vi "DoCollision.vi"(8 "error in (no error)":errorcluster, 10 "GameObject in":refnum<class "GameObject.lvclass">, 11 "Object in":refnum<class "GameObject.lvclass">) -> (0 "error out":errorcluster, 1 "Collided?":bool, 2 "GameObject out":refnum<class "GameObject.lvclass">, 3 "Object out":refnum<class "GameObject.lvclass">)   [LabVIEW 2019, in "RT_Game.lvlib" / "GameObject.lvclass"]
uses:
  GameObject.lvclass
  GameObject.lvclass/GameObject.ctl
  Globals.vi
  RT_Game.lvlib
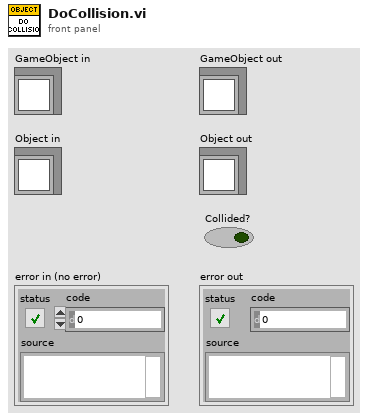
[diagram p1: front panel]
types:
  T1 = typedef "RT_Game.lvlib/Velocity.ctl" = cluster{"x":dbl, "y":dbl}
  T2 = typedef "RT_Game.lvlib/Game.lvclass/Coordinate.ctl" = cluster{"x":dbl, "y":dbl}
  T3 = typedef "RT_Game.lvlib/Direction.ctl" = enum16{"none", "Both", "left", "right", "up", "down"}
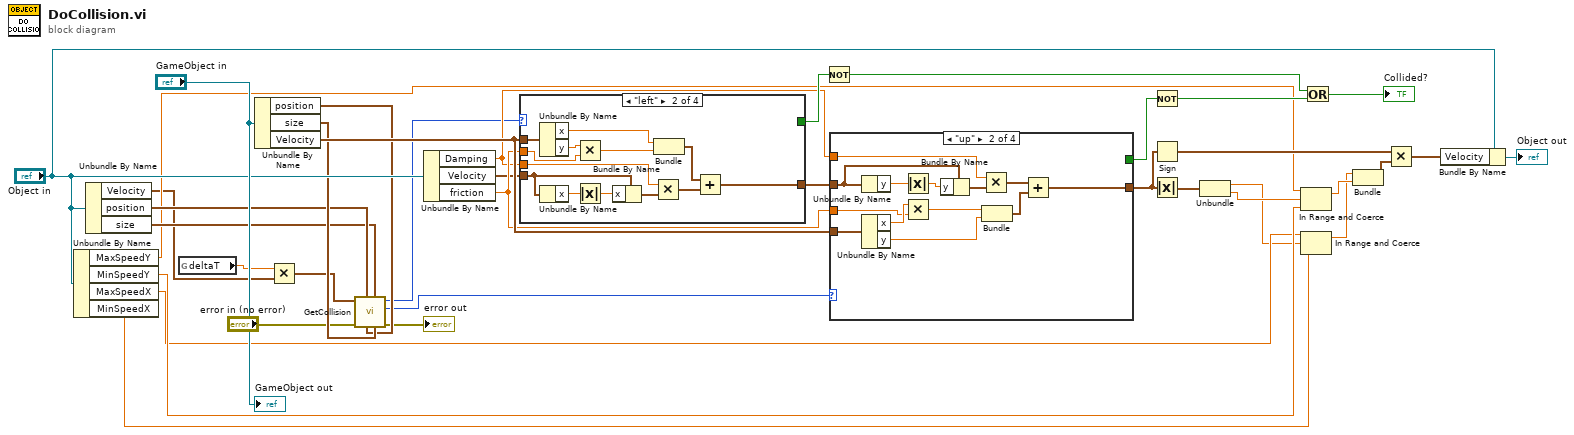
[diagram p0: block diagram]
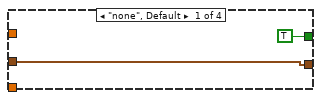
[diagram p2: hidden frame]
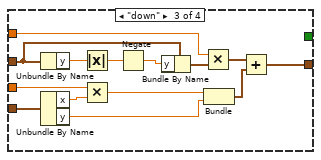
[diagram p3: hidden frame]
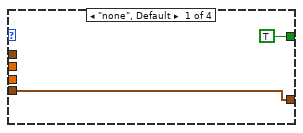
[diagram p5: hidden frame]
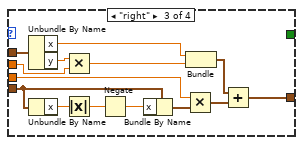
[diagram p6: hidden frame]
diagram:
  n1 = Unbundle By Name("Object in") -> ("MaxSpeedY"=w18:dbl, "MinSpeedY"=w17:dbl, "MaxSpeedX"=w6:dbl, "MinSpeedX"=w5:dbl)
  n2 = Unbundle By Name("Object in") -> ("Velocity"=w10:T1, "position"=w26:T2, "size"=w25:T2)
  n3 = global read "Globals.vi" "deltaT"() -> (w11:dbl)
  n4 = Unbundle By Name("GameObject in") -> ("position"=w27:T2, "size"=w28:T2, "Velocity"=w29:T1)
  n5 = Multiply(x=w11, y=w10) -> (x*y=w16:T1)
  n6 = call "GetCollision.vi"("TheirSize"=w28, "MySize"=w25, "TheirPosition"=w27, "MyPosition"=w26, "error in (no error)"="error in (no error)", "Velocity"=w16) -> ("error out"=→"error out":errorcluster, "direction_y"=w14:T3, "direction_x"=w13:T3)  [unwired: 3 in]
  n7 = Unbundle By Name("Object in") -> ("Damping"=w21:dbl, "Velocity"=w15:T1, "friction"=w22:dbl)
  n8 = case shown="\"left\"" w13 {
    tunnel: w15 -> [w39 w48 w62 w67]
    tunnel: [w39 w50 w64 w67] -> w23
    tunnel: w29 -> [_ w52 w66 _]
    tunnel: w21 -> [_ w44 w58 _]
    tunnel: w22 -> [_ w40 w53 _]
    tunnel: [TRUE _ _ _] -> w30
    frame "none", Default {
    }
    frame "left" {
      n9 = Unbundle By Name(w52) -> ("x"=w46:dbl, "y"=w42:dbl)
      n10 = Unbundle By Name(w48) -> ("x"=w47:dbl)
      n11 = Multiply(x=w42, y=w40) -> (x*y=w41:dbl)
      n12 = Absolute Value(x=w47) -> (abs(x)=w43:dbl)
      n13 = Bundle By Name(cluster=w48, "x"=w43) -> (w49:T1)
      n14 = Multiply(x=w44, y=w49) -> (x*y=w45:T1)
      n15 = Bundle("x"=w46, w41) -> (w51:cluster{"x":dbl, dbl})  [unwired: 1 in]
      n16 = Add(x=w51, y=w45) -> (x+y=w50:T1)
    }
    frame "right" {
      n17 = Unbundle By Name(w66) -> ("x"=w60:dbl, "y"=w55:dbl)
      n18 = Unbundle By Name(w62) -> ("x"=w61:dbl)
      n19 = Multiply(x=w55, y=w53) -> (x*y=w54:dbl)
      n20 = Absolute Value(x=w61) -> (abs(x)=w57:dbl)
      n21 = Negate(x=w57) -> (-x=w56:dbl)
      n22 = Bundle By Name(cluster=w62, "x"=w56) -> (w63:T1)
      n23 = Multiply(x=w58, y=w63) -> (x*y=w59:T1)
      n24 = Bundle("x"=w60, w54) -> (w65:cluster{"x":dbl, dbl})  [unwired: 1 in]
      n25 = Add(x=w65, y=w59) -> (x+y=w64:T1)
    }
    frame "Both" {
    }
  }
  n26 = Not(x=w30) -> (.not. x?=w34:bool)
  n27 = case shown="\"up\"" w14 {
    tunnel: w23 -> [w69 w77 w91 w97]
    tunnel: [w69 w79 w93 w97] -> w19
    tunnel: w29 -> [_ w81 w95 _]
    tunnel: w21 -> [_ w73 w86 _]
    tunnel: w22 -> [_ w71 w83 _]
    tunnel: [TRUE _ _ _] -> w31
    frame "none", Default {
    }
    frame "up" {
      n28 = Unbundle By Name(w77) -> ("y"=w78:dbl)
      n29 = Unbundle By Name(w81) -> ("x"=w72:dbl, "y"=w80:dbl)
      n30 = Absolute Value(x=w78) -> (abs(x)=w74:dbl)
      n31 = Multiply(x=w72, y=w71) -> (x*y=w70:dbl)
      n32 = Bundle By Name(cluster=w77, "y"=w74) -> (w75:T1)
      n33 = Multiply(x=w73, y=w75) -> (x*y=w76:T1)
      n34 = Bundle(w70, "y"=w80) -> (w82:cluster{dbl, "y":dbl})  [unwired: 1 in]
      n35 = Add(x=w76, y=w82) -> (x+y=w79:T1)
    }
    frame "down" {
      n36 = Unbundle By Name(w91) -> ("y"=w92:dbl)
      n37 = Unbundle By Name(w95) -> ("x"=w85:dbl, "y"=w94:dbl)
      n38 = Absolute Value(x=w92) -> (abs(x)=w88:dbl)
      n39 = Multiply(x=w83, y=w85) -> (x*y=w84:dbl)
      n40 = Negate(x=w88) -> (-x=w87:dbl)
      n41 = Bundle By Name(cluster=w91, "y"=w87) -> (w89:T1)
      n42 = Multiply(x=w86, y=w89) -> (x*y=w90:T1)
      n43 = Bundle(w84, "y"=w94) -> (w96:cluster{dbl, "y":dbl})  [unwired: 1 in]
      n44 = Add(x=w90, y=w96) -> (x+y=w93:T1)
    }
    frame "Both" {
    }
  }
  n45 = Not(x=w31) -> (.not. x?=w32:bool)
  n46 = Sign(1:w19) -> (0:w20:T1)
  n47 = Absolute Value(x=w19) -> (abs(x)=w8:T1)
  n48 = Unbundle(w8) -> ("x"=w2:dbl, "y"=w4:dbl)
  n49 = In Range and Coerce(upper limit=w18, x=w4, lower limit=w17) -> (coerced(x)=w7:dbl)  [unwired: 1 out]
  n50 = In Range and Coerce(upper limit=w6, x=w2, lower limit=w5) -> (coerced(x)=w3:dbl)  [unwired: 1 out]
  n51 = Or(x=w34, y=w32) -> (x .or. y?=→"Collided?":bool)
  n52 = Bundle("MaxSpeedX"=w3, "MaxSpeedY"=w7) -> (w1:cluster{"MaxSpeedX":dbl, "MaxSpeedY":dbl})  [unwired: 1 in]
  n53 = Multiply(x=w20, y=w1) -> (x*y=w24:T1)
  n54 = Bundle By Name(cluster="Object in", "Velocity"=w24) -> (→"Object out":refnum<class "GameObject.lvclass">)
  "GameObject out" <- "GameObject in"
